vi "List Directory.vi"(6 "timeout (ms)":i32=30000, 8 "error in (no error)":errorcluster, 10 "remote path":string, 11 "session in":refnum<class "Session.lvclass">) -> (0 "error out":errorcluster, 2 "files and directories":refnum<class "File Attributes.lvclass">[](array[class]), 3 "session out":refnum<class "Session.lvclass">)   [LabVIEW 2020, in "NI_SFTP.lvlib"]
doc: "Returns information about the contents of a remote directory."
uses:
  <vilib>/net/SFTP/NI_SFTP.lvlib
  <vilib>/net/SFTP/Session/Session.lvclass
  <vilib>/net/SFTP/File Attributes/File Attributes.lvclass
  <vilib>/net/SFTP/File Attributes/File Attributes.lvclass/File Attributes.ctl
  <vilib>/Utility/Deadline/NI_Deadline.lvlib
  <vilib>/net/SFTP/API/Support/Command/SSH_FXP_OPENDIR/SSH_FXP_OPENDIR.lvclass
  <vilib>/net/SFTP/API/Support/Command/SSH_FXP_READDIR/SSH_FXP_READDIR.lvclass
  <vilib>/net/SFTP/API/Support/Command/SSH_FXP_CLOSE/SSH_FXP_CLOSE.lvclass
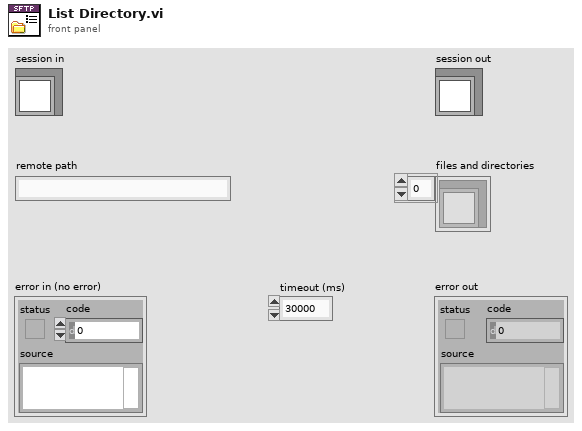
[diagram p1: front panel]
types:
  T1 = typedef "NI_Deadline.lvlib/Deadline.ctl" = cluster{"mode":T2, "deadline (ms)":u32}
  T2 = typedef "NI_Deadline.lvlib/Mode.ctl" = enum16{"Relative", "Use deadline", "Wait forever", "Nonblocking", "N/A"}
  T3 = typedef "NI_SFTP.lvlib/Session.lvclass/Handle.ctl" = u8[]
  T4 = typedef "NI_SFTP.lvlib/Name.ctl" = cluster{"file name":string, "long name":string, "file attributes":T5}
  T5 = typedef "NI_SFTP.lvlib/File Attributes.ctl" = cluster{"SSH_FILEXFER_ATTR_SIZE":bool, "size":u64, "SSH_FILEXFER_ATTR_UIDGID":bool, "uid":u32, "gid":u32, "SSH_FILEXFER_ATTR_PERMISSIONS":bool, "permissions":u32, "SSH_FILEXFER_ATTR_ACMODTIME":bool, "atime":u32, "mtime":u32, "extended":map{string, string}}
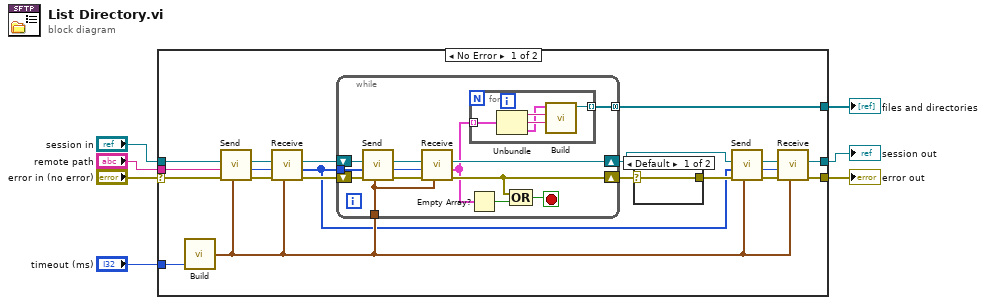
[diagram p0: block diagram]
diagram:
  n1 = case shown="No Error" "error in (no error)" {
    selector: "error in (no error)" -> [w23 w48]
    tunnel: [w22 w48] -> w6
    tunnel: [w8 w47] -> w4
    tunnel: "session in" -> [w14 w47]
    tunnel: "timeout (ms)" -> [w27 _]
    tunnel: "remote path" -> [w15 _]
    tunnel: [w18 _] -> w1
    frame No Error {
      n2 = call <vilib>:"Build.vi"("timeout (ms)"=w27) -> ("Deadline out"=w21:T1)  [unwired: 2 in]
      n3 = call <vilib>:"Send.vi"("Timeout"=w21, "error in"=w23, "filename"=w15, "session in"=w14) -> ("error out"=w26:errorcluster, "request id"=w13:u32, "session out"=w19:refnum<class "Session.lvclass">)  [unwired: 4 in, 1 out]
      n4 = call <vilib>:"Receive.vi"("deadline"=w21, "error in"=w26, "request id"=w13, "session in"=w19) -> ("error out"=w25:errorcluster, "handle"=w10:T3, "session out"=w12:refnum<class "Session.lvclass">)  [unwired: 4 in, 1 out]
      n5 = while {
        shift-right: [w35] -> w17
        shift-left: w25 -> [w41]
        tunnel: w21 -> [w39]
        tunnel: [w37] -> w18 mode=concatenating
        shift-right: [w32] -> w11
        shift-left: w12 -> [w33]
        tunnel: w10 -> [w29]
        stop <- w36 stop-if-true
        n6 = call <vilib>:"Send.vi"("Timeout"=w39, "error in"=w41, "handle"=w29, "session in"=w33) -> ("error out"=w40:errorcluster, "request id"=w30:u32, "session out"=w38:refnum<class "Session.lvclass">)  [unwired: 4 in, 1 out]
        n7 = call <vilib>:"Receive.vi"("Timeout"=w39, "error in"=w40, "request id"=w30, "session in"=w38) -> ("error out"=w35:errorcluster, "files"=w31:T4[], "session out"=w32:refnum<class "Session.lvclass">)  [unwired: 4 in, 1 out]
        n8 = Empty Array?(array=w31) -> (empty?=w34:bool)
        n9 = for {
          tunnel: w31 -> [w46] mode=indexing
          tunnel: [w42] -> w37 mode=indexing
          n10 = Unbundle(w46) -> ("file name"=w45:string, "long name"=w44:string, "file attributes"=w43:T5)
          n11 = call <vilib>:"Build.vi"("long name"=w44, "file name"=w45, "file attributes"=w43) -> ("file attributes out"=w42:refnum<class "File Attributes.lvclass">)  [unwired: 8 in]
        }
        n12 = Compound Arithmetic op=OR(w35, w34) -> (w36:bool)
      }
      n13 = case shown="Default" w17 {
        selector: w17 -> [w28 _]
        tunnel: [w28 _] -> w16
        frame #0 {
        }
        frame #1 {
        }
      }
      n14 = call <vilib>:"Send.vi"("deadline"=w21, "error in"=w16, "handle"=w10, "session in"=w11) -> ("error out"=w24:errorcluster, "request id"=w9:u32, "session out"=w20:refnum<class "Session.lvclass">)  [unwired: 4 in, 1 out]
      n15 = call <vilib>:"Receive.vi"("deadline"=w21, "error in"=w24, "request id"=w9, "session in"=w20) -> ("error out"=w22:errorcluster, "session out"=w8:refnum<class "Session.lvclass">)  [unwired: 4 in, 2 out]
    }
    frame Error {
    }
  }
  "error out" <- w6
  "session out" <- w4
  "files and directories" <- w1
